vi "Check and Log Plugin Timeout Error.vi"(6 "-1014 timeout (ms)":u32=10000, 8 "New Error":errorcluster, 10 "Previous Error":errorcluster, 11 "CIF_UI in":refnum<class "CIF_UI.lvclass">) -> (0 "error out":errorcluster)   [LabVIEW 2021, in "CIF_UI.lvclass"]
doc: "This error management and logging VI is intended to run in the timeout case of the event structure in plugin UI loops. It will manage the registration of new local errors by checking if a previous, uncleared, error exists.\n\nIt will also mute specific errors and check for use cases where the plugin should shutdown automatically."
uses:
  CIF_UI.lvclass
  CIF_UI.lvclass/CIF_UI.ctl
  Utilities/Get Human Readable Error.vi
  <vilib>/CIF Foundation/CIF Utilities/Errors/Append Error Location.vi
  <vilib>/CIF Foundation/CIF Utilities/Errors/Human Readable Error Message.vi
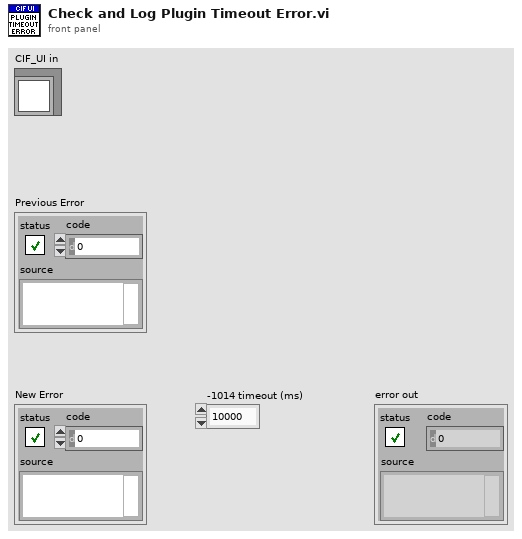
[diagram p1: front panel]
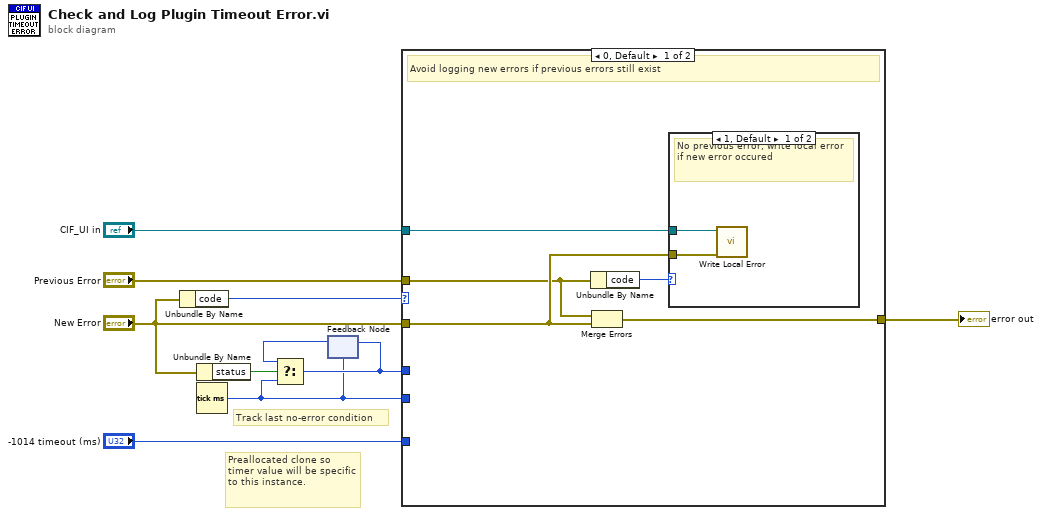
[diagram p0: block diagram]
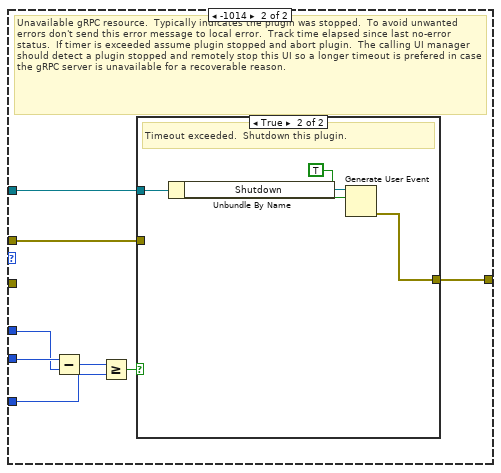
[diagram p3: hidden frame]
diagram:
  # "Preallocated clone so timer value will be specific to this instance."
  # "Track last no-error condition"
  n1 = Unbundle By Name("New Error") -> ("code"=w7:i32)
  n2 = Unbundle By Name("New Error") -> ("status"=w5:bool)
  n3 = Tick Count (ms)() -> (millisecond timer value=w2:u32)
  n4 = feedback #1(w2) -> (w4:u32)
  n5 = Select(t=w4, s=w5, f=w2) -> (s? t:f=w3:u32)
  n6 = feedback-in #1(w3) -> ()
  n7 = case shown="0, Default" w7 {
    tunnel: "Previous Error" -> [w12 w19]
    tunnel: [w15 w20] -> w9
    tunnel: "CIF_UI in" -> [w14 w18]
    tunnel: "New Error" -> [w13 _]
    tunnel: w3 -> [_ w24]
    tunnel: w2 -> [_ w25]
    tunnel: "-1014 timeout (ms)" -> [_ w22]
    frame 0, Default {
      # "Avoid logging new errors if previous errors still exist"
      n8 = Unbundle By Name(w12) -> ("code"=w11:i32)
      n9 = Merge Errors(w12, w13) -> (w15:errorcluster)
      n10 = case shown="1, Default" w11 {
        tunnel: w14 -> [w17 _]
        tunnel: w13 -> [w16 _]
        frame 1, Default {
          # "No previous error, write local error if new error occured"
          n11 = call "Write Local Error.vi"("error in (no error)"=w16, "CIF_UI in"=w17) -> ()  [unwired: 9 in, 1 out]
        }
        frame 0 {
        }
      }
    }
    frame -1014 {
      # "Unavailable gRPC resource.  Typically indicates the plugin was stopped.  To avoid unwanted errors don't send this error message to local error.  Track time elapsed since last no-error status.  If timer is exceeded assume plugin stopped and abort plugin.  The calling UI manager should detect a plugin stopped and remotely stop this UI so a longer timeout is prefered in case the gRPC server is unavailable for a recoverable reason."
      n12 = Subtract(x=w25, y=w24) -> (x-y=w23:u32)
      n13 = Greater Or Equal?(x=w23, y=w22) -> (x >= y?=w21:bool)
      n14 = case shown="True" w21 {
        tunnel: [w26 w28] -> w20
        tunnel: w19 -> [w26 _]
        tunnel: w18 -> [_ w27]
        frame False {
          # "Timeout has not expired.  Mute error and continue"
        }
        frame True {
          # "Timeout exceeded.  Shutdown this plugin."
          n15 = Unbundle By Name(w27) -> ("Shutdown"=w30:refnum<user-event>)
          n16 = Generate User Event(user event=w30, event data cluster=TRUE ("event data")) -> (error out=w28:errorcluster)  [unwired: 2 in, 1 out]
        }
      }
    }
  }
  "error out" <- w9
